vi "Rx FIFOs switch.vi"(0 "rx.data sink":enum16{"SFP Port 0", "SFP Port 1", "Host"}(ring)=enum."SFP Port 1") -> ()   [LabVIEW 2016]
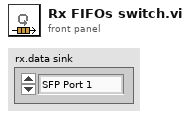
[diagram p1: front panel]
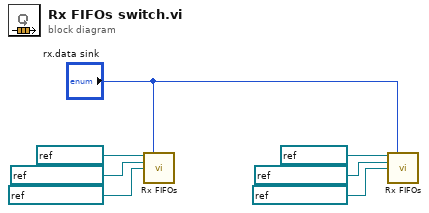
[diagram p0: block diagram]
diagram:
  n1 = call "Rx FIFOs.vi"("rx.fifo"=refnum<k21> "rx 0.fifo", "rx.data sink"="rx.data sink", "rx.host fifo"=refnum<k21> "rx 0.host fifo", "rx.sfp fifo"=refnum<k21> "rx 0.sfp 0 fifo") -> ()  [unwired: 12 in]
  n2 = call "Rx FIFOs.vi"("rx.fifo"=refnum<k21> "rx 1.fifo", "rx.data sink"="rx.data sink", "rx.host fifo"=refnum<k21> "rx 1.host fifo", "rx.sfp fifo"=refnum<k21> "rx 1.sfp 1 fifo") -> ()  [unwired: 12 in]
